vi "Write NET_HttpResponseTask.vi"(8 "error in (no error)":errorcluster, 10 "NET_HttpResponseMessage":refnum<k24>, 11 "HttpResponseMessage in":refnum<class "HttpResponseMessage.lvclass">) -> (0 "error out":errorcluster, 3 "HttpResponseMessage out":refnum<class "HttpResponseMessage.lvclass">)   [LabVIEW 2018, in "HttpClient_NET.lvlib" / "HttpResponseMessage.lvclass"]
doc: "<b> </b> <b> </b>\nHttpClient_NET\nJustin Young - Viviota\nCopyright (c) 2021\nLicense: BSD"
uses:
  HttpResponseMessage.lvclass
  HttpResponseMessage.lvclass/HttpResponseMessage.ctl
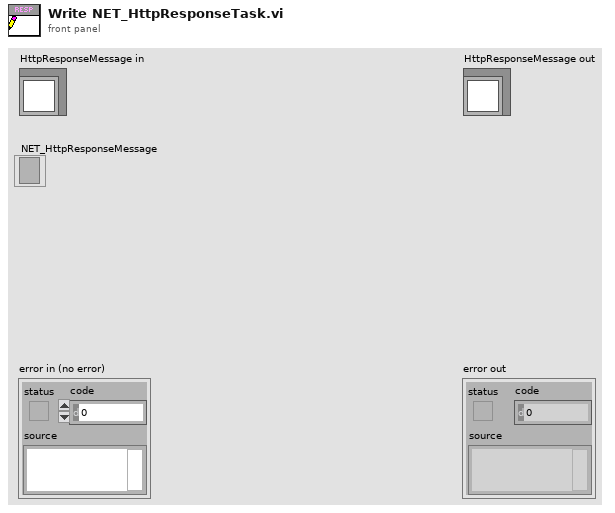
[diagram p1: front panel]
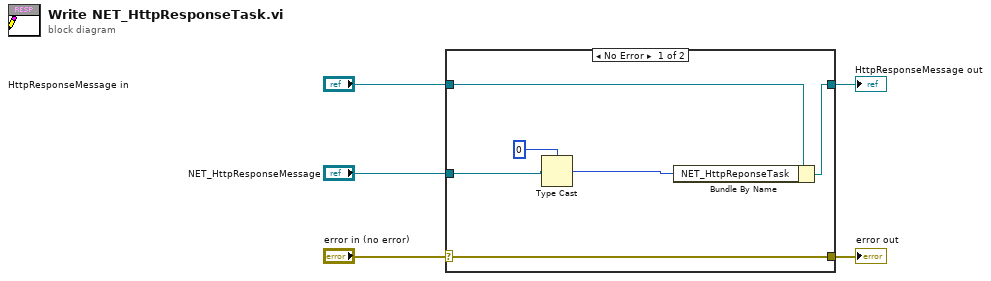
[diagram p0: block diagram]
diagram:
  n1 = case shown="No Error" "error in (no error)" {
    selector: "error in (no error)" -> [w11 w12]
    tunnel: [w11 w12] -> w4
    tunnel: [w9 w13] -> w2
    tunnel: "HttpResponseMessage in" -> [w10 w13]
    tunnel: "NET_HttpResponseMessage" -> [w8 _]
    frame No Error {
      n2 = Type Cast(type=i64 0 ("NET_HttpReponseMessage"), x=w8) -> (*(type *) &x=w6:i64)
      n3 = Bundle By Name(cluster=w10, "NET_HttpReponseTask"=w6) -> (w9:refnum<class "HttpResponseMessage.lvclass">)
    }
    frame Error {
    }
  }
  "error out" <- w4
  "HttpResponseMessage out" <- w2
